vi "ChangeField v0.80.vi"(0 "Starting Field (T)":dbl format="%.2f", 1 "Tolerance (T)":dbl=0.0151 min=0.0001 max=1.0 step=0.0001 format="%.3f", 2 "Desired Field (T)":dbl format="%.2f", 3 "SweepRate (T/min)":dbl=10.0 format="%.2f", 5 "error in (no error)":errorcluster) -> (4 "Status":cluster{bool, bool, "Ramp Status":u16, bool}, 6 "Tesla":dbl(knob) caption="Current Field (T)" scale=0.002325024974988211..1.2000000000000002 scale format="%.1f", 7 "Cell":string, 8 "error out":errorcluster)   [LabVIEW 2019]
uses:
  Globals and TypeDefs/Global Varibal Control.vi
panel:
  in  "stop":bool
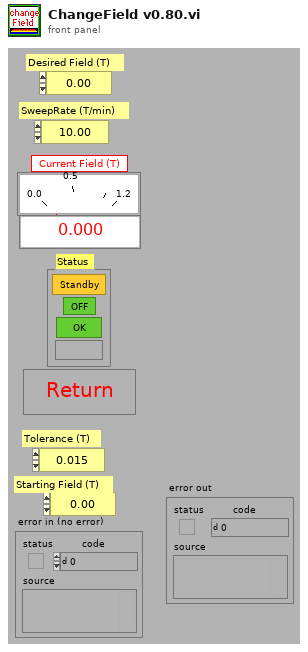
[diagram p1: front panel]
types:
  T1 = cluster{"PS on/off":bool, "PS fault?":bool, "Ramp Status":u16, "PS Control?":bool}
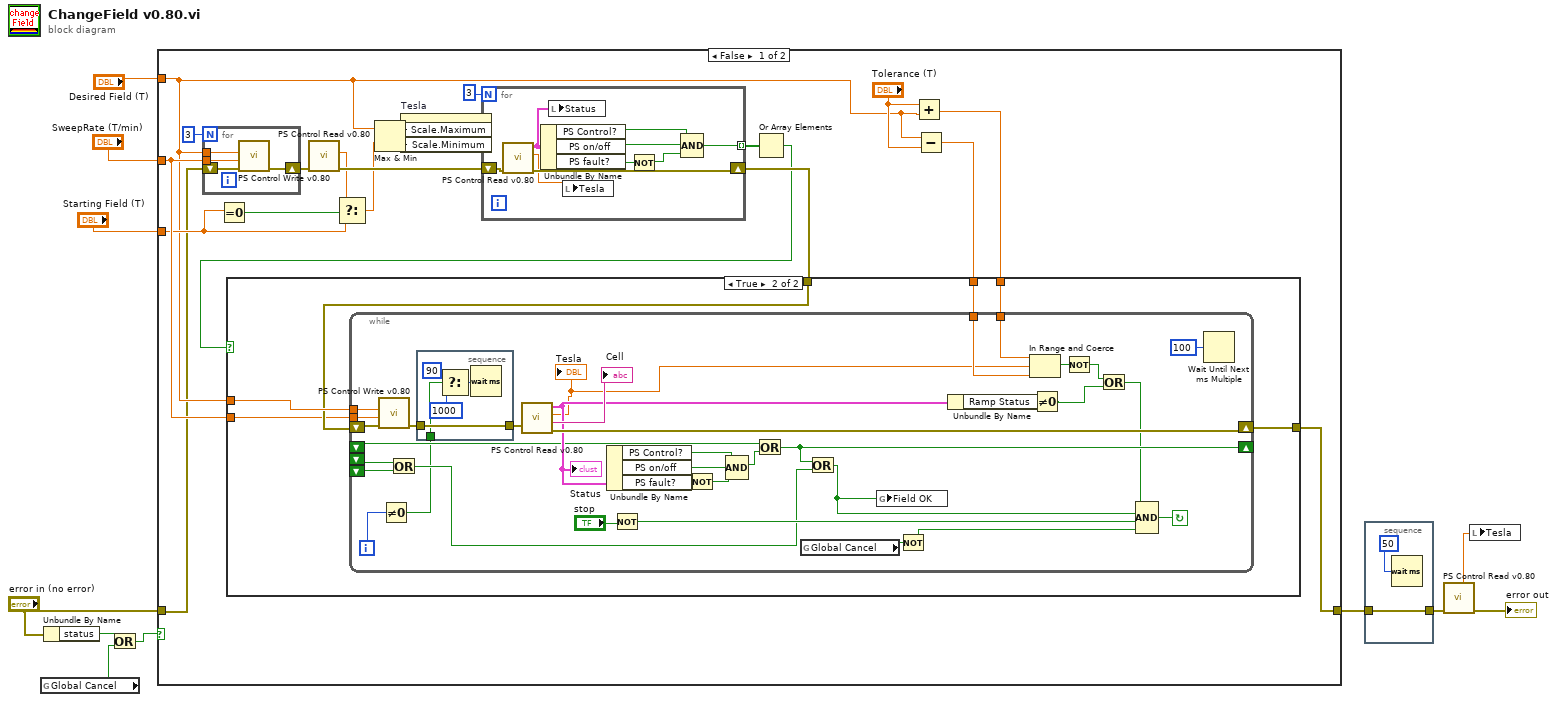
[diagram p0: block diagram]
diagram:
  n1 = global read "Global Varibal Control.vi" "Global Cancel"() -> (w1:bool)
  n2 = Unbundle By Name("error in (no error)") -> ("status"=w9:bool)
  n3 = Or(x=w9, y=w1) -> (x .or. y?=w10:bool)
  n4 = case shown="False" w10 {
    tunnel: "error in (no error)" -> [w13 w92]
    tunnel: [w25 w92] -> w6
    tunnel: "SweepRate (T/min)" -> [w21 _]
    tunnel: "Desired Field (T)" -> [w15 _]
    tunnel: "Starting Field (T)" -> [w18 _]
    frame False {
      n5 = for {
        N: 3 -> [_]
        tunnel: w21 -> [w35]
        tunnel: w15 -> [w34]
        shift-right: [w32] -> w12
        shift-left: w13 -> [w33]
        n6 = call "PS Control Write v0.80.vi"("error in (no error)"=w33, "Slew Rate"=w35, "Setpoint"=w34) -> ("error out"=w32:errorcluster)  [unwired: 7 in, 1 out]
      }
      n7 = Equal To 0?(x=w18) -> (x = 0?=w19:bool)
      n8 = call "PS Control Read v0.80.vi"("error in (no error)"=w12) -> ("error out"=w20:errorcluster, "Current"=w17:dbl)  [unwired: 3 in, 3 out]
      n9 = Select(t=w17, s=w19, f=w18) -> (s? t:f=w16:dbl)
      n10 = Max & Min(x=w15, y=w16) -> (max(x,y)=w29:dbl, min(x,y)=w28:dbl)
      n11 = property on="Tesla" class="Knob (strict)"("Scale.Maximum"=w29, "Scale.Minimum"=w28) -> ()  [unwired: 2 in, 2 out]
      n12 = for {
        N: 3 -> [_]
        tunnel: [w89] -> w30 mode=indexing
        shift-right: [w88] -> w27
        shift-left: w20 -> [w87]
        n13 = call "PS Control Read v0.80.vi"("error in (no error)"=w87) -> ("error out"=w88:errorcluster, "Current"=w83:dbl, "Status"=w86:T1)  [unwired: 3 in, 2 out]
        n14 = Unbundle By Name(w86) -> ("PS Control?"=w85:bool, "PS on/off"=w84:bool, "PS fault?"=w91:bool)
        n15 = local write "Status"(w86) -> ()
        n16 = local write "Tesla"(w83) -> ()
        n17 = Not(x=w91) -> (.not. x?=w90:bool)
        n18 = Compound Arithmetic op=AND(w85, w84, w90) -> (w89:bool)
      }
      n19 = Or Array Elements(Boolean array=w30) -> (logical OR=w26:bool)
      n20 = Add(x="Tolerance (T)", y=w15) -> (x+y=w23:dbl)
      n21 = Subtract(x=w15, y="Tolerance (T)") -> (x-y=w22:dbl)
      n22 = case shown="True" w26 {
        tunnel: w15 -> [_ w42]
        tunnel: w27 -> [w36 w41]
        tunnel: [w36 w40] -> w25
        tunnel: w23 -> [_ w39]
        tunnel: w22 -> [_ w38]
        tunnel: w21 -> [_ w37]
        frame False {
        }
        frame True {
          n23 = while {
            tunnel: w38 -> [w50]
            tunnel: w39 -> [w51]
            shift-left: _ -> [w61]
            shift-left: _ -> [w62]
            shift-left: _ -> [w67]
            shift-right: [w60] -> _
            shift-left: w41 -> [w74]
            shift-right: [w75] -> w40
            tunnel: w37 -> [w76]
            tunnel: w42 -> [w77]
            i -> [w53]
            stop <- w65 continue-if-true
            n24 = call "PS Control Write v0.80.vi"("error in (no error)"=w74, "Slew Rate"=w76, "Setpoint"=w77) -> ("error out"=w55:errorcluster)  [unwired: 7 in, 1 out]
            n25 = Not Equal To 0?(x=w53) -> (x != 0?=w52:bool)
            n26 = Or(x=w62, y=w61) -> (x .or. y?=w59:bool)
            n27 = stacked-sequence {
              tunnel: [w82] -> w54
              tunnel: w55 -> [w82]
              tunnel: w52 -> [w81]
              frame #0 {
                n28 = Select(t=90, s=w81, f=u32 1000 ("millisecond multiple")) -> (s? t:f=w79:u32)
                n29 = Wait (ms)(milliseconds to wait=w79) -> ()  [unwired: 1 out]
              }
            }
            n30 = call "PS Control Read v0.80.vi"("error in (no error)"=w54) -> ("error out"=w75:errorcluster, "Cell"=→"Cell":string, "Current"=w49:dbl, "Status"=w71:T1)  [unwired: 3 in, 1 out]
            "Status" <- w71
            "Tesla" <- w49
            n31 = Unbundle By Name(w71) -> ("PS Control?"=w57:bool, "PS on/off"=w56:bool, "PS fault?"=w70:bool)
            n32 = Not(x="stop") -> (.not. x?=w63:bool)
            n33 = Not(x=w70) -> (.not. x?=w69:bool)
            n34 = Compound Arithmetic op=AND(w57, w56, w69) -> (w68:bool)
            n35 = Or(x=w67, y=w68) -> (x .or. y?=w60:bool)
            n36 = global read "Global Varibal Control.vi" "Global Cancel"() -> (w48:bool)
            n37 = Or(x=w60, y=w59) -> (x .or. y?=w47:bool)
            n38 = global write "Global Varibal Control.vi" "Field OK"(w47) -> ()
            n39 = Not(x=w48) -> (.not. x?=w58:bool)
            n40 = Unbundle By Name(w71) -> ("Ramp Status"=w73:u16)
            n41 = In Range and Coerce(upper limit=w51, x=w49, lower limit=w50) -> (In Range?=w46:bool)  [unwired: 1 out]
            n42 = Not Equal To 0?(x=w73) -> (x != 0?=w45:bool)
            n43 = Not(x=w46) -> (.not. x?=w43:bool)
            n44 = Or(x=w43, y=w45) -> (x .or. y?=w44:bool)
            n45 = Compound Arithmetic op=AND(w44, w47, w63, w58) -> (w65:bool)
            n46 = Wait Until Next ms Multiple(millisecond multiple=u32 100) -> ()  [unwired: 1 out]
          }
        }
      }
    }
    frame True {
    }
  }
  n47 = stacked-sequence {
    tunnel: [w94] -> w5
    tunnel: w6 -> [w94]
    frame #0 {
      n48 = Wait (ms)(milliseconds to wait=u32 50) -> ()  [unwired: 1 out]
    }
  }
  n49 = call "PS Control Read v0.80.vi"("error in (no error)"=w5) -> ("error out"=→"error out":errorcluster, "Current"=w7:dbl)  [unwired: 3 in, 3 out]
  n50 = local write "Tesla"(w7) -> ()
